vi "elog global.vi"() -> ()   [LabVIEW 2022 SP3]
panel:
  in  "Elog Init":T1={"Complete Path Elog Exec"="C:\\Software\\CTS\\support.vi\\elog\\elog lib", "IP Address Server Elog"="192.168.149.102", "Port Server Elog"="8080"}
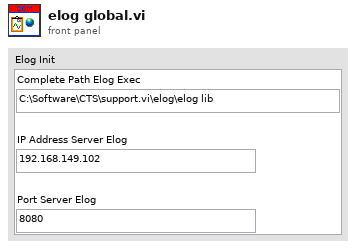
[diagram p1: front panel]
types:
  T1 = cluster{"Complete Path Elog Exec":string, "IP Address Server Elog":string, "Port Server Elog":string}
diagram:
